vi "Update DataBase.vi"(4 "Cost":u8, 6 "Name":string, 8 "error in (no error)":errorcluster, 9 "Datetime string":string, 10 "Database path":path, 11 "Contabilidad in":refnum<class "Contabilidad.lvclass">) -> (0 "error out":errorcluster, 3 "Contabilidad out":refnum<class "Contabilidad.lvclass">)   [LabVIEW 2020, in "Contabilidad.lvlib" / "Contabilidad.lvclass"]
uses:
  Contabilidad.lvclass
  <vilib>/drjdpowell/SQLite Library/SQL Connection/Open (path).vi
  <vilib>/drjdpowell/SQLite Library/SQL Connection/Open (string).vi
  <vilib>/AdvancedString/Path To Command Line String.vi
  <vilib>/drjdpowell/SQLite Library/SQL Connection/Execute SQL (No results).vi
  <vilib>/drjdpowell/SQLite Library/SQL Connection/Connection.lvclass
  <vilib>/drjdpowell/SQLite Library/SQLite.lvlib
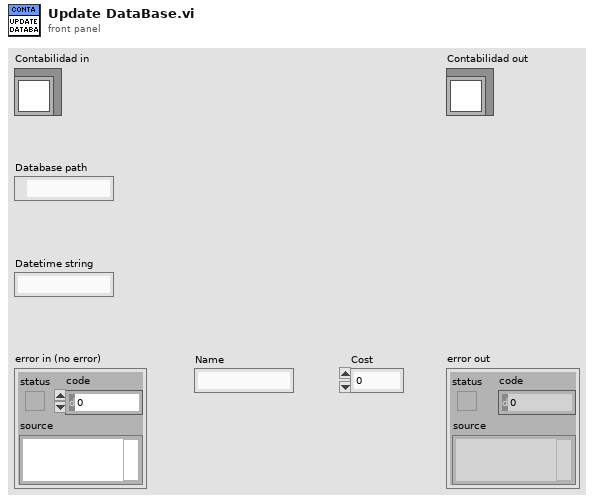
[diagram p1: front panel]
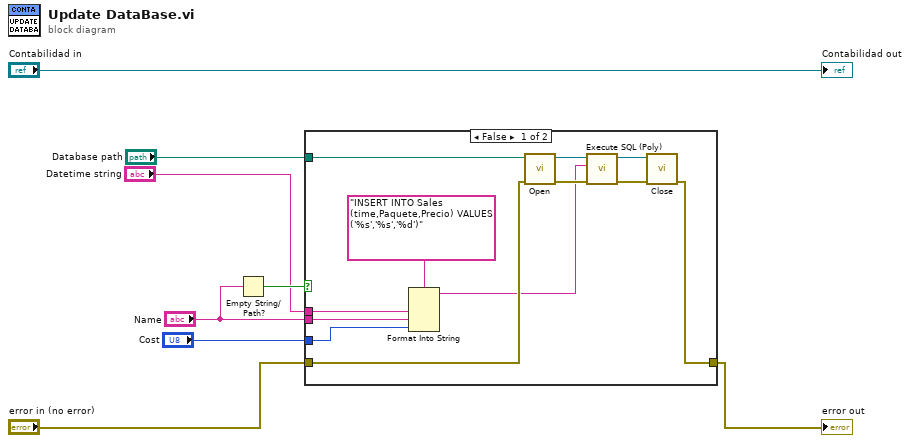
[diagram p0: block diagram]
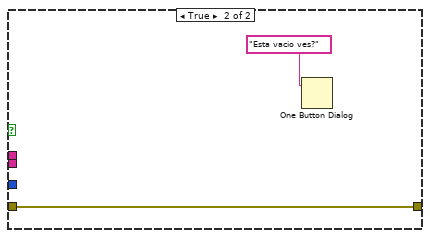
[diagram p2: hidden frame]
diagram:
  n1 = Empty String/Path?(string/path="Name") -> (empty?=w7:bool)
  n2 = case shown="False" w7 {
    tunnel: "Database path" -> [w20 _]
    tunnel: "error in (no error)" -> [w17 w21]
    tunnel: [w16 w21] -> w4
    tunnel: "Datetime string" -> [w11 _]
    tunnel: "Name" -> [w10 _]
    tunnel: "Cost" -> [w9 _]
    frame False {
      n3 = Format Into String(format string="INSERT INTO Sales (time,Paquete,Precio) VALUES ('%s','%s','%d')", w11, w10, w9) -> (resulting string=w13:string)  [unwired: 2 in, 1 out]
      n4 = call-poly <vilib>:"Open.vi"("error in (no error)"=w17, "db file"=w20) -> ("error out"=w14:errorcluster, "SQLite Connection"=w19:refnum<class "Connection.lvclass">)  [unwired: 8 in]
      n5 = call-poly <vilib>:"Execute SQL (Poly).vi"("error in (no error)"=w14, "SQL"=w13, "SQLite Connection in"=w19) -> ("error out"=w15:errorcluster, "SQLite Connection"=w18:refnum<class "Connection.lvclass">)  [unwired: 7 in]
      n6 = call-dynamic "Close.vi"("error in (no error)"=w15, "SQLite Connection in"=w18) -> ("error out"=w16:errorcluster)  [unwired: 9 in]
    }
    frame True {
      n7 = One Button Dialog(message="Esta vacio ves?") -> ()  [unwired: 1 in, 1 out]
    }
  }
  "error out" <- w4
  "Contabilidad out" <- "Contabilidad in"
